vi "Test.vi"(8 "error in (no error)":errorcluster, 10 "board image":T1, 11 "GPIB Board Design in":refnum<class "GPIB Board Design.lvclass">) -> (0 "error out":errorcluster, 2 "pass?":T2, 3 "Test name":string)   [LabVIEW 2018, in "GPIB Board Design.lvclass"]
doc: "Image check for blocks that are common to all types of boards."
uses:
  GPIB Board Design.lvclass
  Common/Pass Fail Boolean.ctl
  Common/Board Image.ctl
  Board Design_class/Board Design.lvclass
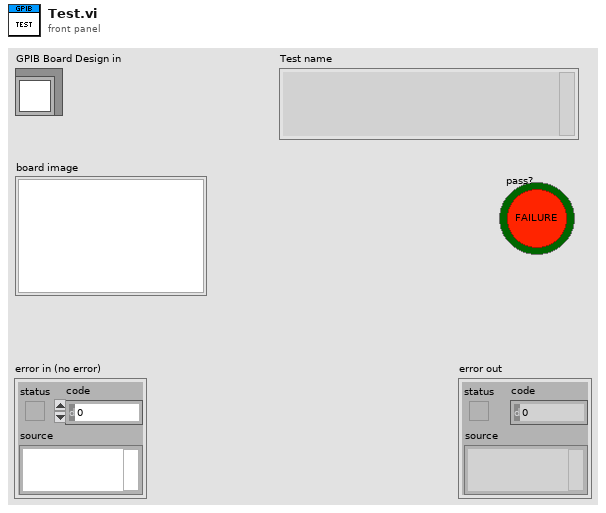
[diagram p1: front panel]
types:
  T1 = typedef "Board Image.ctl" = picture
  T2 = typedef "Pass Fail Boolean.ctl" = bool
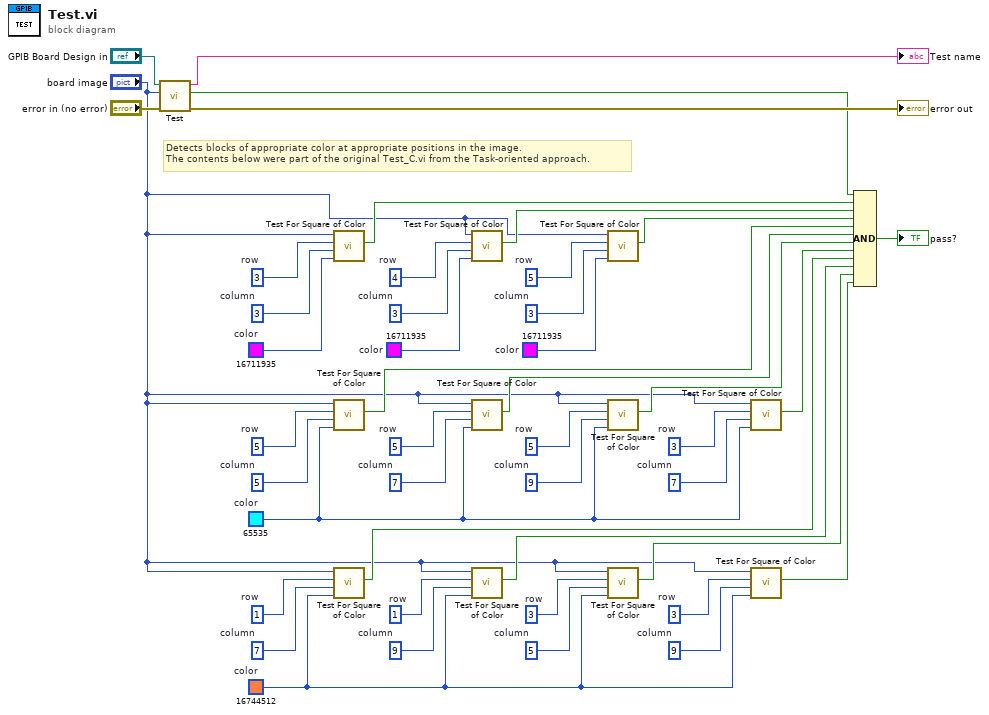
[diagram p0: block diagram]
diagram:
  w6 = i16 9  # column
  w7 = i16 3  # row
  w11 = i16 7  # column
  w10 = i16 3  # row
  w16 = i16 5  # column
  w15 = i16 3  # row
  w17 = i16 9  # column
  w18 = i16 1  # row
  w20 = i16 7  # column
  w19 = i16 1  # row
  w5 = u32 16744512  # color
  w30 = i16 9  # column
  w31 = i16 5  # row
  w29 = i16 7  # column
  w28 = i16 5  # row
  w26 = i16 5  # column
  w27 = i16 5  # row
  w9 = u32 65535  # color
  w33 = i16 3  # column
  w32 = i16 5  # row
  w34 = u32 16711935  # color
  w36 = i16 3  # column
  w37 = i16 4  # row
  w35 = u32 16711935  # color
  w40 = i16 3  # column
  w39 = i16 3  # row
  w41 = u32 16711935  # color
  # "Detects blocks of appropriate color at appropriate positions in the image.\nThe contents below were part of the original Test_C.vi from the Task-oriented approach."
  n1 = call-parent "Test.vi"("error in (no error)"="error in (no error)", "board image"="board image", "Board Design in"="GPIB Board Design in") -> ("error out"=→"error out":errorcluster, "pass?"=w2:T2, "Test name"=→"Test name":string)  [unwired: 6 in]
  n2 = call "Test For Square of Color.vi"("color"=w41, "column"=w40, "row"=w39, "board image"="board image") -> ("pass?"=w38:T2)  [unwired: 7 in]
  n3 = call "Test For Square of Color.vi"("color"=w9, "column"=w26, "row"=w27, "board image"="board image") -> ("pass?"=w23:T2)  [unwired: 7 in]
  n4 = call "Test For Square of Color.vi"("color"=w5, "column"=w20, "row"=w19, "board image"="board image") -> ("pass?"=w12:T2)  [unwired: 7 in]
  n5 = call "Test For Square of Color.vi"("color"=w35, "column"=w36, "row"=w37, "board image"="board image") -> ("pass?"=w25:T2)  [unwired: 7 in]
  n6 = call "Test For Square of Color.vi"("color"=w9, "column"=w29, "row"=w28, "board image"="board image") -> ("pass?"=w22:T2)  [unwired: 7 in]
  n7 = call "Test For Square of Color.vi"("color"=w5, "column"=w17, "row"=w18, "board image"="board image") -> ("pass?"=w13:T2)  [unwired: 7 in]
  n8 = call "Test For Square of Color.vi"("color"=w34, "column"=w33, "row"=w32, "board image"="board image") -> ("pass?"=w24:T2)  [unwired: 7 in]
  n9 = call "Test For Square of Color.vi"("color"=w9, "column"=w30, "row"=w31, "board image"="board image") -> ("pass?"=w21:T2)  [unwired: 7 in]
  n10 = call "Test For Square of Color.vi"("color"=w5, "column"=w16, "row"=w15, "board image"="board image") -> ("pass?"=w14:T2)  [unwired: 7 in]
  n11 = call "Test For Square of Color.vi"("color"=w9, "column"=w11, "row"=w10, "board image"="board image") -> ("pass?"=w8:T2)  [unwired: 7 in]
  n12 = call "Test For Square of Color.vi"("color"=w5, "column"=w6, "row"=w7, "board image"="board image") -> ("pass?"=w4:T2)  [unwired: 7 in]
  n13 = Compound Arithmetic op=AND(w2, w38, w25, w24, w23, w22, w21, w8, w12, w13, w14, w4) -> (→"pass?":T2)
